vi "receiveData_DiagnosticVersion.vi"(8 "error in (no error)":errorcluster, 11 "ILC in":refnum<class "ILC.lvclass">) -> (0 "error out":errorcluster, 3 "ILC out":refnum<class "ILC.lvclass">)   [LabVIEW 2013, in "ILCCommon.lvlib" / "ILC.lvclass"]
uses:
  <userlib>/Common/ILC/ILC/ILC.lvclass
  <userlib>/Common/ILC/ILC/ILC.lvclass/ILC.ctl
  <userlib>/Common/SerialProtocols/SerialCommunicator/SerialCommunicator.lvclass
panel:
  out "appended array":string[](array[string])
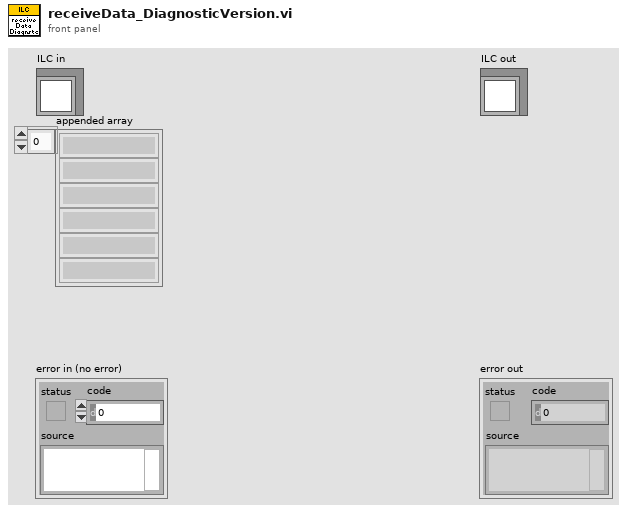
[diagram p1: front panel]
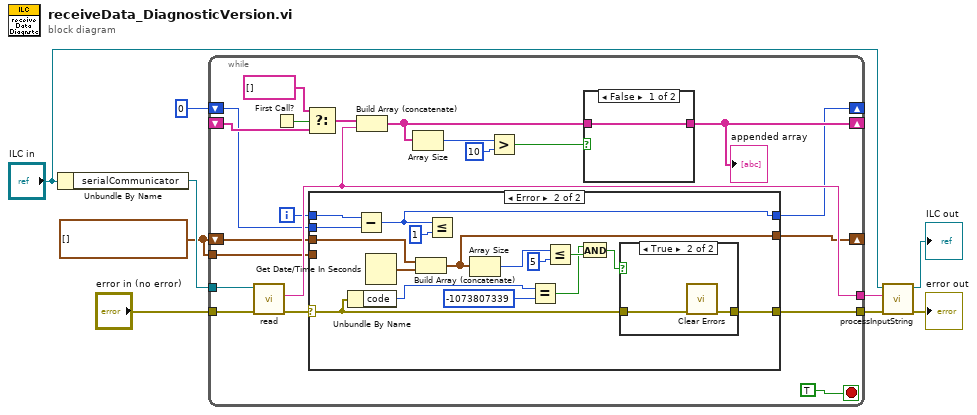
[diagram p0: block diagram]
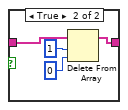
[diagram p4: hidden frame]
diagram:
  w1 = timestamp[] []
  n1 = Unbundle By Name("ILC in") -> ("serialCommunicator"=w8:refnum<class "SerialCommunicator.lvclass">)
  n2 = while {
    tunnel: [w16] -> w9
    tunnel: w8 -> [w30]
    tunnel: "error in (no error)" -> [w29]
    shift-right: [w18] -> _
    shift-left: _ -> [w24]
    tunnel: [w27] -> w3
    shift-right: [w14] -> _
    shift-left: 0 -> [w13]
    shift-right: [w12] -> _
    shift-left: w1 -> [w11]
    tunnel: w1 -> [w10]
    i -> [w15]
    stop <- TRUE stop-if-true
    n3 = call-dynamic "read.vi"("error in (no error)"=w29, "SerialCommunicator in"=w30) -> ("error out"=w17:errorcluster, "stringRead"=w27:string)  [unwired: 7 in, 1 out]
    n4 = First Call?() -> (First Call?: T/F=w26:bool)
    n5 = Select(t=string[] [], s=w26, f=w24) -> (s? t:f=w23:string[])
    n6 = case shown="Error" w17 {
      selector: w17 -> [w33 w47]
      tunnel: [w33 w46] -> w16
      tunnel: w15 -> [w32 w45]
      tunnel: [w32 w43] -> w14
      tunnel: w13 -> [_ w44]
      tunnel: [w31 w39] -> w12
      tunnel: w11 -> [_ w40]
      tunnel: w10 -> [w31 _]
      frame No Error {
      }
      frame Error {
        n7 = Unbundle By Name(w47) -> ("code"=w49:i32)
        n8 = Subtract(x=w45, y=w44) -> (x-y=w43:i32)
        n9 = Get Date/Time In Seconds() -> (seconds since 1Jan1904=w41:timestamp)
        n10 = Build Array (concatenate)(w40, w41) -> (w39:timestamp[])
        n11 = Less Or Equal?(x=w43, y=1) -> ()  [unwired: 1 out]
        n12 = Array Size(array=w39) -> (size(s)=w38:i32)
        n13 = Equal?(x=w49, y=-1073807339) -> (x = y?=w35:bool)
        n14 = Less Or Equal?(x=w38, y=5) -> (x <= y?=w36:bool)
        n15 = And(x=w35, y=w36) -> (x .and. y?=w34:bool)
        n16 = case shown="True" w34 {
          tunnel: w47 -> [w50 w52]
          tunnel: [w50 w51] -> w46
          frame False {
          }
          frame True {
            n17 = call <vilib>:"Clear Errors.vi"("error in (no error)"=w52) -> ("error out"=w51:errorcluster)  [unwired: 6 in]
          }
        }
      }
    }
    n18 = Build Array (concatenate)(w23, w27) -> (w19:string[])
    n19 = Array Size(array=w19) -> (size(s)=w22:i32)
    n20 = Greater?(x=w22, y=10) -> (0:w20:bool)
    n21 = case shown="False" w20 {
      tunnel: w19 -> [w53 w57]
      tunnel: [w53 w54] -> w18
      frame False {
      }
      frame True {
        n22 = Delete From Array(array=w57, length=1, index=0) -> (array with subset deleted=w54:string[])  [unwired: 1 out]
      }
    }
    "appended array" <- w18
  }
  n23 = call <userlib>:"processInputString.vi"("error in (no error)"=w9, "stringRead"=w3, "ILC in"="ILC in") -> ("error out"=→"error out":errorcluster, "ILC out"=→"ILC out":refnum<class "ILC.lvclass">)  [unwired: 7 in]
